vi "Configure Voltage.vi"(0 "VISA resource name":refnum<visa-resource-name>, 1 "Voltage Mode (0: Fixed)":i32(ring) items=["Fixed", "Step", "Pulse", "List"], 5 "Voltage Auto Level Control (0: On)":u16(ring) items=["On", "Off", "Regulation"], 7 "Voltage Source (0:Internal)":u16(ring) items=["Internal", "External"], 9 "Voltage Level (0V)":dbl, 11 "error in (no error)":errorcluster, 12 "Transient Voltage Level (0V)":dbl, 13 "Voltage Protection Range (150V)":u16(ring)=150 items=["150"=150, "300"=300]) -> (4 "VISA resource name out":refnum<visa-resource-name>, 15 "error out":errorcluster)   [LabVIEW 2014, in "Cal Inst.lvlib" / "California Instruments iX Series.lvlib"]
doc: "Configures the output voltage of the AC source."
uses:
  California Instruments iX Series.lvlib
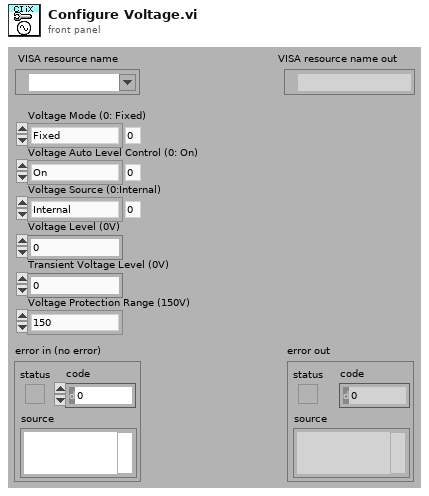
[diagram p1: front panel]
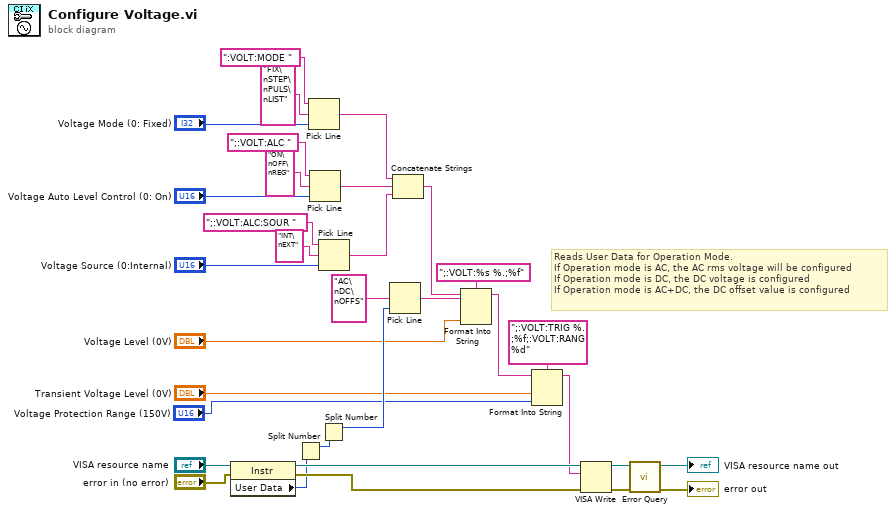
[diagram p0: block diagram]
diagram:
  # "Reads User Data for Operation Mode. \nIf Operation mode is AC, the AC rms voltage will be configured\nIf Operation mode is DC, the DC voltage is configured\nIf Operation mode is AC+DC, the DC offset value is configured"
  n1 = property class="Instr"(reference="VISA resource name", error in="error in (no error)") -> (reference out=w15:refnum<visa-resource-name>, error out=w14:errorcluster, "User Data"=w13:u32)
  n2 = Split Number(x=w13) -> (hi(x)=w12:u16)  [unwired: 1 out]
  n3 = Pick Line(string ("")=":VOLT:MODE ", multi-line string="FIX\nSTEP\nPULS\nLIST", line index="Voltage Mode (0: Fixed)") -> (output string=w23:string)
  n4 = Pick Line(string ("")=";:VOLT:ALC ", multi-line string="ON\nOFF\nREG", line index="Voltage Auto Level Control (0: On)") -> (output string=w22:string)
  n5 = Pick Line(string ("")=";:VOLT:ALC:SOUR ", multi-line string="INT\nEXT", line index="Voltage Source (0:Internal)") -> (output string=w18:string)
  n6 = Split Number(x=w12) -> (hi(x)=w10:u8)  [unwired: 1 out]
  n7 = Pick Line(multi-line string="AC\nDC\nOFFS", line index=w10) -> (output string=w9:string)  [unwired: 1 in]
  n8 = Concatenate Strings(w23, w22, w18) -> (w7:string)
  n9 = Format Into String(format string=";:VOLT:%s %.;%f", initial string=w7, w9, "Voltage Level (0V)") -> (resulting string=w5:string)  [unwired: 1 in, 1 out]
  n10 = Format Into String(format string=";:VOLT:TRIG %.;%f;:VOLT:RANG %d", initial string=w5, "Transient Voltage Level (0V)", "Voltage Protection Range (150V)") -> (resulting string=w2:string)  [unwired: 1 in, 1 out]
  n11 = VISA Write(VISA resource name=w15, write buffer=w2, error in (no error)=w14) -> (VISA resource name out=w31:refnum<visa-resource-name>, error out=w30:errorcluster)  [unwired: 1 out]
  n12 = call "Error Query.vi"("error in (no error)"=w30, "VISA resource name"=w31) -> ("error out"=→"error out":errorcluster, "VISA resource name out"=→"VISA resource name out":refnum<visa-resource-name>)  [unwired: 6 in, 2 out]
